vi "Create or Replace File.vi"(8 "error in (no error)":errorcluster, 10 "Log File Base Path":path) -> (0 "error out":errorcluster, 2 "File Path":path, 3 "Refnum out":refnum<k34>)   [LabVIEW 2019, in "Logger.lvlib"]
doc: "_____\nBased on DQMH Project Template 6.0.0.91."
uses:
  Logger.lvlib
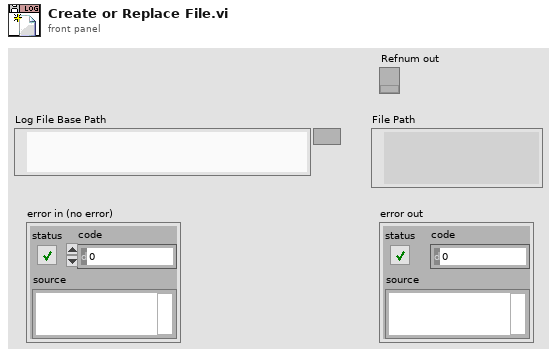
[diagram p1: front panel]
types:
  T1 = enum16{"open", "open or create", "create or replace", "create", "open (read-only)"}
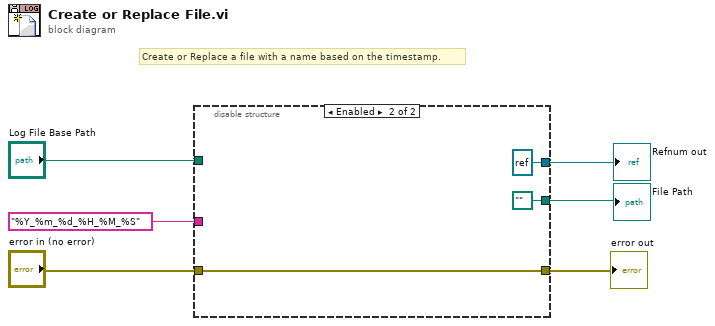
[diagram p0: block diagram]
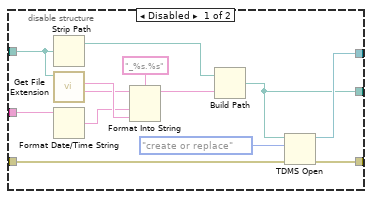
[diagram p2: hidden frame]
diagram:
  # "Create or Replace a file with a name based on the timestamp."
  n1 = disable-structure shown="Enabled" {
    disable-tunnel: "error in (no error)" -> [w19 w20]
    disable-tunnel: [w18 refnum<k34> refnum ("Refnum out")] -> w5
    disable-tunnel: [w16 w20] -> w4
    disable-tunnel: "%Y_%m_%d_%H_%M_%S" -> [w9 _]
    disable-tunnel: "Log File Base Path" -> [w8 _]
    disable-tunnel: [w7 path "" ("File Path")] -> w1
    frame Disabled {
      n2 = Strip Path(path=w8) -> (stripped path=w11:path)  [unwired: 1 out]
      n3 = call <vilib>:"Get File Extension.vi"("file"=w8) -> ("filename without extension"=w10:string, "lowercase file extension"=w14:string)  [unwired: 6 in, 3 out]
      n4 = Format Date/Time String(time format string (%c)=w9) -> (date/time string=w13:string)  [unwired: 2 in]
      n5 = Format Into String(format string="_%s.%s", initial string=w10, w13, w14) -> (resulting string=w15:string)  [unwired: 1 in, 1 out]
      n6 = Build Path(base path=w11, name or relative path=w15) -> (appended path=w7:path)
      n7 = TDMS Open(8:w19, 10:T1."create or replace" ("operation (0:open)"), 11:w7) -> (0:w16:errorcluster, 3:w18:refnum<k34>)  [unwired: 4 in]
    }
    frame Enabled {
    }
  }
  "Refnum out" <- w5
  "error out" <- w4
  "File Path" <- w1
